vi "save_time.vi"(4 "input time":timestamp) -> (0 "Puls Width":string, 1 "last time":timestamp, 2 "is Big Energy":bool)   [LabVIEW 2018]
uses:
  <vilib>/Utility/miscctls.llb/LVDateTimeRec.ctl
  <vilib>/Utility/file.llb/Write Delimited Spreadsheet (string).vi
panel:
  out "x-y":dbl
  out "Plus Width":dbl
  out "last_txt":string
  out "大小":i32
  out "文件名":string[](array[string])
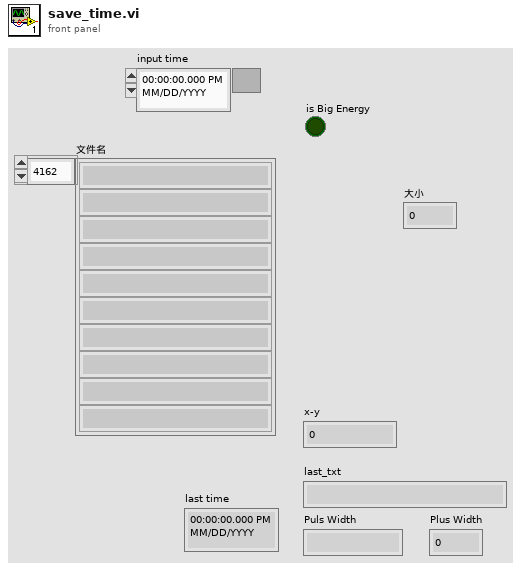
[diagram p1: front panel]
types:
  T1 = typedef "LVDateTimeRec.ctl" = cluster{"fractional second":dbl, "second":i32, "minute":i32, "hour":i32, "day of month":i32, "month":i32, "year":i32, "day of week":i32, "day of year":i32, "DST":i32}
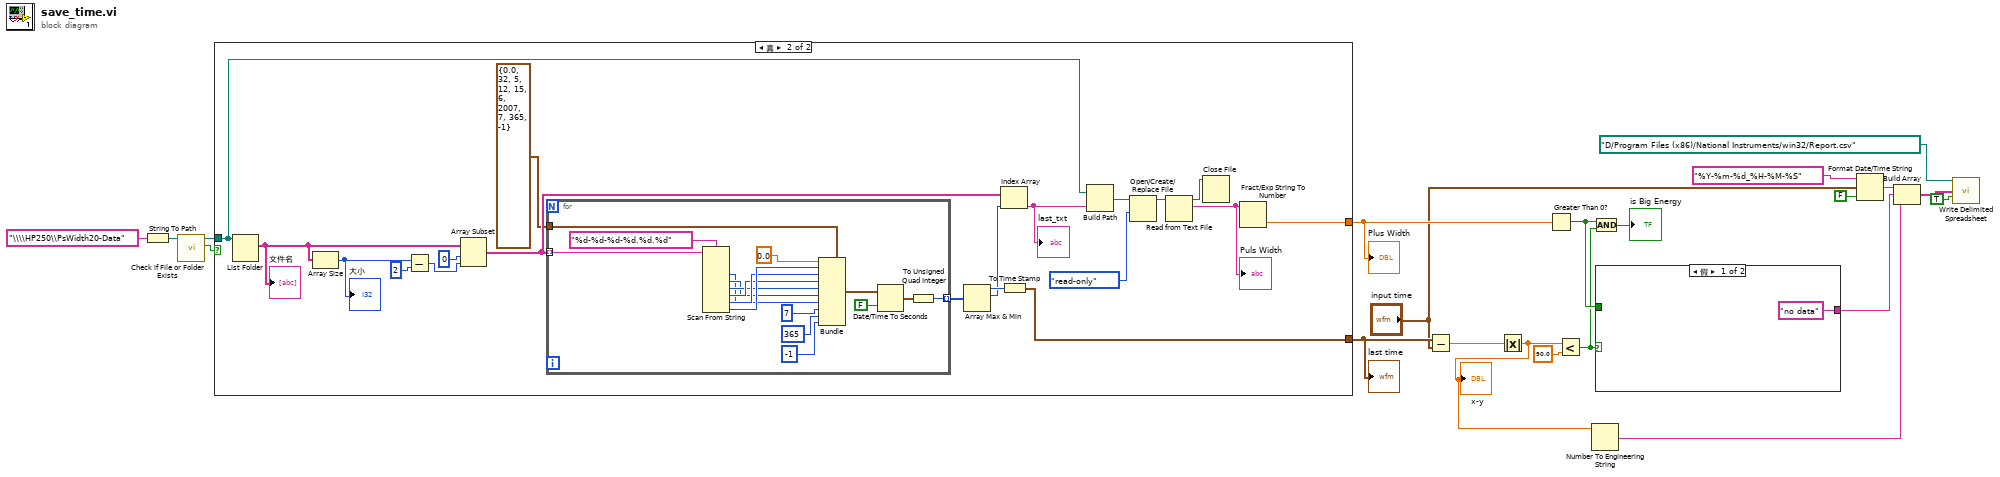
[diagram p0: block diagram]
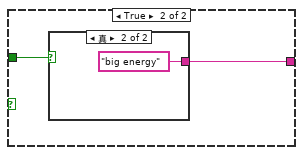
[diagram p2: hidden frame]
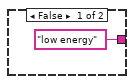
[diagram p3: hidden frame]
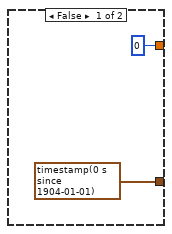
[diagram p4: hidden frame]
diagram:
  n1 = String To Path(string="\\\\HP250\\PsWidth20-Data") -> (path=w20:path)
  n2 = call <vilib>:"Check if File or Folder Exists.vi"("path"=w20) -> ("file or folder exists?"=w18:bool, "dup path"=w19:path)  [unwired: 8 in, 1 out]
  n3 = case shown="真" w18 {
    tunnel: w19 -> [_ w26]
    tunnel: [0 w25] -> w15
    tunnel: [timestamp(0 s since 1904-01-01) w24] -> w17
    frame False {
    }
    frame True {
      n4 = List Folder(path=w26) -> (filenames=w42:string[])  [unwired: 3 in, 3 out]
      "文件名" <- w42
      n5 = Array Size(array=w42) -> (size(s)=w40:i32)
      "大小" <- w40
      n6 = Subtract(x=w40, y=2) -> (x-y=w38:i32)
      n7 = Array Subset(array=w42, index=0 ("索引"), length=w38) -> (w35:string[])
      n8 = for {
        tunnel: w35 -> [w46] mode=indexing
        tunnel: [w44] -> w37 mode=indexing
        tunnel: T1 {"fractional second"=0.0, "second"=32, "minute"=5, "hour"=12, "day of month"=15, "month"=6, "year"=2007, "day of week"=7, "day of year"=365, "DST"=-1} ("日期时间记录") -> [w43]
        n9 = Scan From String(format string="%d-%d-%d-%d.%d.%d" ("格式字符串"), input string=w46) -> (output 1=w53:i32, output 2=w54:i32, output 3=w55:i32, output 4=w56:i32, output 5=w57:i32, output 6=w58:i32)  [unwired: 8 in, 3 out]
        n10 = Bundle(cluster=w43, "fractional second"=0.0, "second"=w58, "minute"=w57, "hour"=w56, "day of month"=w55, "month"=w54, "year"=w53, "day of week"=7, "day of year"=365, "DST"=-1) -> (w49:T1)
        n11 = Date/Time To Seconds(1:FALSE ("是UTC (F)"), 2:w49) -> (0:w45:timestamp)
        n12 = To Unsigned Quad Integer(1:w45) -> (0:w44:u64)
      }
      n13 = Array Max & Min(array=w37) -> (max value=w36:u64, max index (indices)=w34:i32)  [unwired: 2 out]
      n14 = Index Array(array=w35, index=w34) -> (element=w29:string)
      "last_txt" <- w29
      n15 = To Time Stamp(1:w36) -> (0:w24:timestamp)
      n16 = Build Path(base path=w26, name or relative path=w29) -> (appended path=w28:path)
      n17 = Open/Create/Replace File(file path (use dialog)=w28, access (0:read/write)=enum16{"read/write", "read-only", "write-only"}."read-only" ("权限(0:read/write)")) -> (refnum out=w31:refnum<file>)  [unwired: 4 in, 2 out]
      n18 = Read from Text File(file (use dialog)=w31) -> (refnum out=w30:refnum<file>, text=w27:string)  [unwired: 3 in, 2 out]
      "Puls Width" <- w27
      n19 = Close File(refnum=w30) -> ()  [unwired: 1 in, 2 out]
      n20 = Fract/Exp String To Number(string=w27) -> (number=w25:dbl)  [unwired: 3 in, 1 out]
    }
  }
  "Plus Width" <- w15
  "last time" <- w17
  n21 = Subtract(x=w17, y="input time") -> (x-y=w3:dbl)
  n22 = Absolute Value(x=w3) -> (abs(x)=w2:dbl)
  "x-y" <- w2
  n23 = Greater Than 0?(x=w15) -> (x > 0?=w5:bool)
  n24 = Less?(x=w2, y=90.0) -> (x < y?=w4:bool)
  n25 = Number To Engineering String(4:w2) -> (0:w1:string)  [unwired: 3 in]
  n26 = And(x=w5, y=w4) -> (x .and. y?=→"is Big Energy":bool)
  n27 = case shown="假" w4 {
    tunnel: ["no data" w62] -> w8
    tunnel: w5 -> [_ w61]
    frame False {
    }
    frame True {
      n28 = case shown="真" w61 {
        tunnel: ["low energy" "big energy"] -> w62
        frame False {
        }
        frame True {
        }
      }
    }
  }
  n29 = Format Date/Time String(time format string (%c)="%Y-%m-%d_%H-%M-%S" ("时间格式字符串(%c)"), seconds (now)="input time", UTC format=FALSE ("UTC格式")) -> (date/time string=w9:string)
  n30 = Build Array(w9, w8, w1) -> (w7:string[])
  n31 = call-poly <vilib>:"Write Delimited Spreadsheet.vi"("file path (dialog if empty)"=path "D:/Program Files (x86)/National Instruments/win32/Report.csv", "1D data"=w7, "append to file? (new file:F)"=TRUE) -> ()  [unwired: 11 in, 2 out]
